vi "Slope#2.vi"(0 "Y2":dbl, 5 "Y1":dbl, 7 "X2 (1)":dbl=1.0, 9 "X1":dbl, 11 "error in (no error)":errorcluster) -> (4 "Theta(rad)":dbl, 6 "Theta (degree)":dbl, 8 "Slope (m)":dbl, 15 "error out":errorcluster)   [LabVIEW 2020]
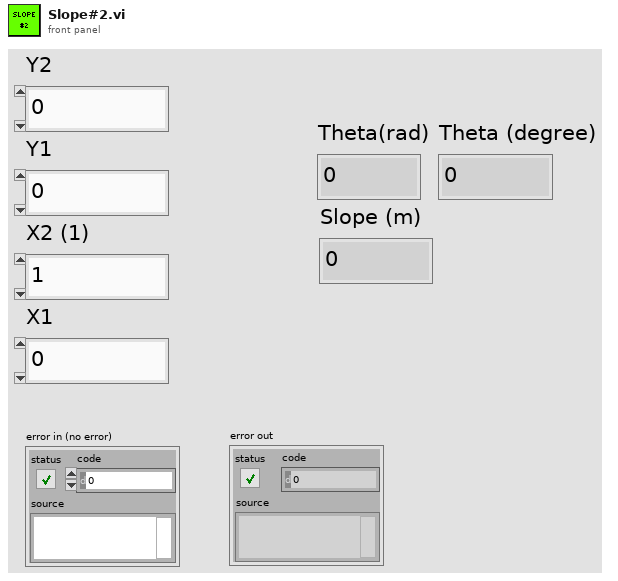
[diagram p1: front panel]
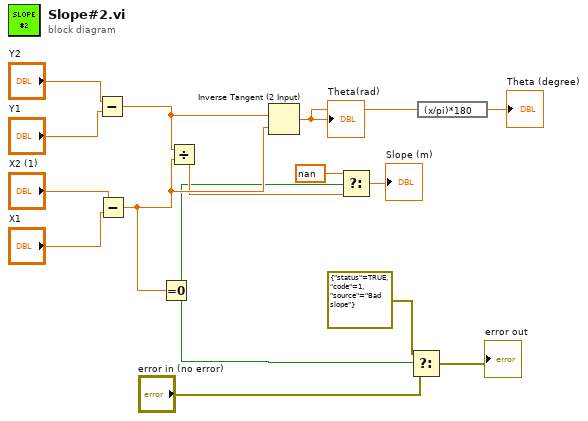
[diagram p0: block diagram]
diagram:
  n1 = Subtract(x="Y2", y="Y1") -> (x-y=w11:dbl)
  n2 = Subtract(x="X2 (1)", y="X1") -> (x-y=w9:dbl)
  n3 = Equal To 0?(x=w9) -> (x = 0?=w3:bool)
  n4 = Divide(x=w11, y=w9) -> (x/y=w5:dbl)
  n5 = Inverse Tangent (2 Input)(1:w9, 2:w11) -> (0:w2:dbl)
  "Theta(rad)" <- w2
  n6 = Select(t=nan, s=w3, f=w5) -> (s? t:f=→"Slope (m)":dbl)
  n7 = Select(t=errorcluster {"status"=TRUE, "code"=1, "source"="Bad slope"} ("error constant"), s=w3, f="error in (no error)") -> (s? t:f=→"error out":errorcluster)
  n8 = expression code="(x/pi)*180"(w2) -> (→"Theta (degree)":dbl)
